vi "Boolean Logic Test.vi"() -> ()   [LabVIEW 2011]
panel:
  in  "stop":bool
  out "Numeric":dbl
  in  "Boolean 4":bool
  in  "Boolean 3":bool
  in  "Boolean 2":bool
  in  "Boolean":bool
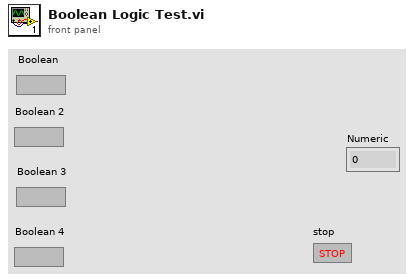
[diagram p1: front panel]
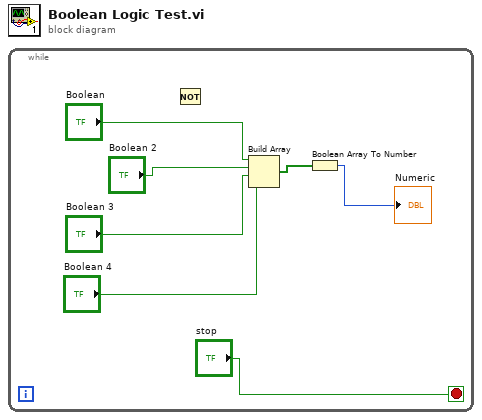
[diagram p0: block diagram]
diagram:
  n1 = while {
    stop <- "stop" stop-if-true
    n2 = Not() -> ()  [unwired: 1 in, 1 out]
    n3 = Build Array("Boolean", "Boolean 2", "Boolean 3", "Boolean 4") -> (w2:bool[])
    n4 = Boolean Array To Number(Boolean array=w2) -> (number=→"Numeric":u32)
  }
